vi "SQLEXEC.vi"(1 "value":dbl, 2 "tag":dbl) -> (0 "Query":string caption="Result")   [LabVIEW 2021]
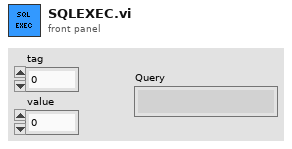
[diagram p1: front panel]
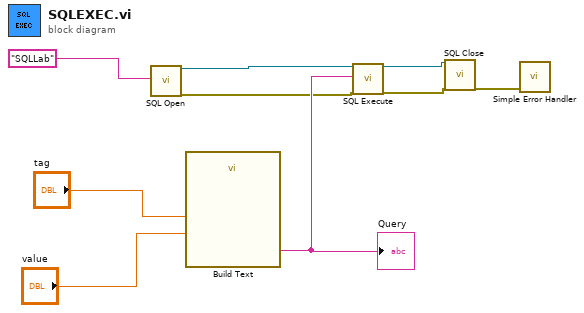
[diagram p0: block diagram]
diagram:
  n1 = call "SQL Open.vi"("ConnectionString In"="SQLLab") -> ("Connection Out"=w8:refnum<k7>, "Error out"=w6:errorcluster)  [unwired: 17 in]
  n2 = call "Build Text"("tag"="tag", "value"="value") -> ("Result"=w7:string)  [unwired: 12 in, 1 out]
  "Query" <- w7
  n3 = call "SQL Execute.vi"("Connection In"=w8, "SQL Query"=w7, "Error in (no error)"=w6) -> ("Connection Out"=w4:refnum<k7>, "Error out"=w3:errorcluster)  [unwired: 15 in]
  n4 = call "SQL Close.vi"("Connection In"=w4, "Error in (no error)"=w3) -> ("Error out"=w5:errorcluster)  [unwired: 17 in]
  n5 = call <vilib>:"Simple Error Handler.vi"("error in (no error)"=w5) -> ()  [unwired: 4 in, 5 out]
